vi "format version as string.vi"(8 "error in":errorcluster, 11 "version":T1) -> (0 "error out":errorcluster, 3 "String":string)   [LabVIEW 2017, in "DSF Configuration Utility.lvlib"]
uses:
  DSF Configuration Utility.lvlib
  DSF Configuration API/1.0.0/Public/Controls/Version Info.ctl
  DSF Configuration API/1.0.0/DSF Configuration API.lvlib
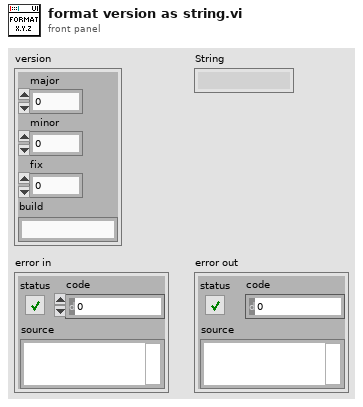
[diagram p1: front panel]
types:
  T1 = typedef "DSF Configuration API.lvlib/Version Info.ctl" = cluster{"major":u32, "minor":u32, "fix":u32, "build":string}
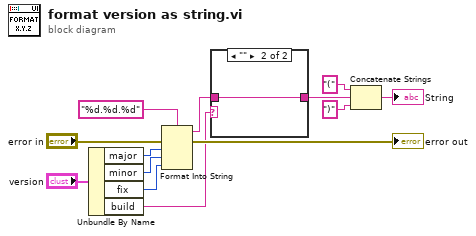
[diagram p0: block diagram]
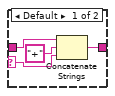
[diagram p2: hidden frame]
diagram:
  n1 = Unbundle By Name("version") -> ("major"=w8:u32, "minor"=w9:u32, "fix"=w10:u32, "build"=w3:string)
  n2 = Format Into String(format string="%d.%d.%d", error in="error in", w8, w9, w10) -> (resulting string=w2:string, error out=→"error out":errorcluster)  [unwired: 1 in]
  n3 = case shown="\"\"" w3 {
    selector: w3 -> [w16 _]
    tunnel: w2 -> [w15 w18]
    tunnel: [w14 w18] -> w1
    frame Default {
      n4 = Concatenate Strings(w15, "+" ("string"), w16) -> (w14:string)
    }
    frame "" {
    }
  }
  n5 = Concatenate Strings("(" ("string"), w1, ")" ("string")) -> (→"String":string)
